vi "BCC.vi"(11 "输入校验十六进制":string) -> (3 "BCC校验结果":string)   [LabVIEW 2017]
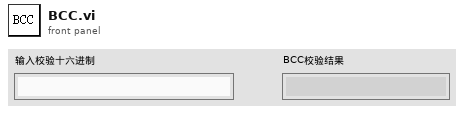
[diagram p1: front panel]
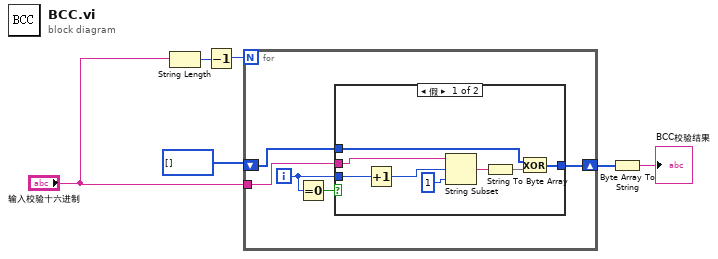
[diagram p0: block diagram]
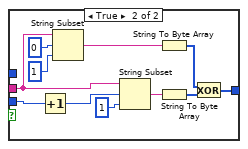
[diagram p2: hidden frame]
diagram:
  n1 = String Length(string="输入校验十六进制") -> (length=w6:i32)
  n2 = Decrement(x=w6) -> (x-1=w5:i32)
  n3 = for {
    N: w5 -> [_]
    tunnel: "输入校验十六进制" -> [w10]
    shift-right: [w7] -> w4
    shift-left: u8[] [] -> [w8]
    i -> [w9]
    n4 = Equal To 0?(x=w9) -> (x = 0?=w11:bool)
    n5 = case shown="假" w11 {
      tunnel: w10 -> [w19 w27]
      tunnel: w9 -> [w18 w25]
      tunnel: [w12 w20] -> w7
      tunnel: w8 -> [w14 _]
      frame False {
        n6 = Increment(x=w18) -> (x+1=w17:i32)
        n7 = String Subset(string=w19, offset (0)=w17, length (rest)=1 ("长度（剩余）")) -> (substring=w15:string)
        n8 = String To Byte Array(string=w15) -> (unsigned byte array=w13:u8[])
        n9 = Exclusive Or(1:w13, 2:w14) -> (0:w12:u8[])
      }
      frame True {
        n10 = Increment(x=w25) -> (x+1=w26:i32)
        n11 = String Subset(string=w27, offset (0)=0 ("偏移量(0)"), length (rest)=1 ("长度（剩余）")) -> (substring=w28:string)
        n12 = String Subset(string=w27, offset (0)=w26, length (rest)=1 ("长度（剩余）")) -> (substring=w23:string)
        n13 = String To Byte Array(string=w28) -> (unsigned byte array=w22:u8[])
        n14 = String To Byte Array(string=w23) -> (unsigned byte array=w21:u8[])
        n15 = Exclusive Or(1:w21, 2:w22) -> (0:w20:u8[])
      }
    }
  }
  n16 = Byte Array To String(unsigned byte array=w4) -> (string=→"BCC校验结果":string)
